vi "JanisDC_3Channel_LKS331_3SRS830.vi"() -> ()   [LabVIEW 2014]
uses:
  <vilib>/Utility/file.llb/Write To Spreadsheet File (DBL).vi
panel:
  out "Probe Temp":dbl format="%.3f"
  out "Cryostat Temp":dbl format="%.3f"
  in  "Tab Control":enum32{"Page 1", "Page 3"}(tab)
  in  "Start T":dbl=130.0
  in  "T Step":dbl=1.0
  in  "End T":dbl
  in  "Mid T":dbl
  in  "T Step 2":dbl=1.0
  in  "Seconds for Stability":dbl=200.0
  in  "SRS830_1\nAddress":i16
  in  "SRS830_2\nAddress":i16
  in  "Save file path":path
  in  "error in (no error)":errorcluster
  out "error out":errorcluster
  in  "Amplitude":dbl=0.75
  in  "Delay Time (s)":dbl=0.4
  in  "Frequency":dbl=0.1
  in  "Offset":dbl=3.0
  in  "Phase":dbl
  in  "Amplifier Offset":dbl=0.1 caption="Frequency"
  in  "Amplifier Gain":dbl=0.1 caption="Frequency"
  in  "LKS331\nAddress":i16
  in  "Setpoint Proximity":dbl=0.01 format="%#.3g"
  in  "Required Stability":dbl=0.002 format="%#.4g"
  in  "SRS830_3\nAddress":i16
  out "XY Graph 3":cluster{dbl, dbl}[](graph) caption="SRS2"
  out "XY Graph 4":cluster{dbl, dbl}[](graph) caption="SRS1"
  out "XY Graph 5":cluster{dbl, dbl}[](graph) caption="LR700"
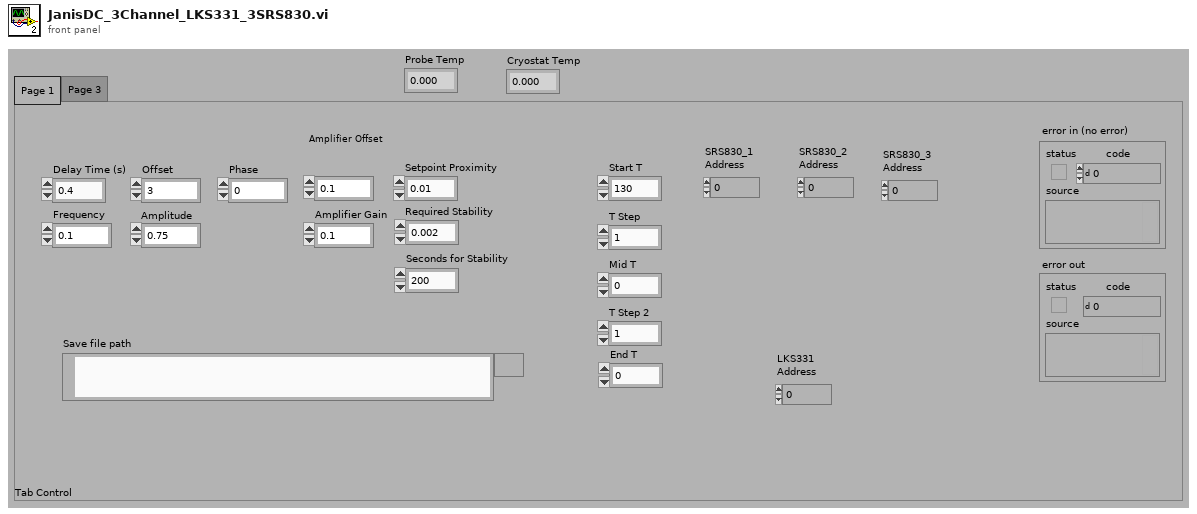
[diagram p1: front panel]
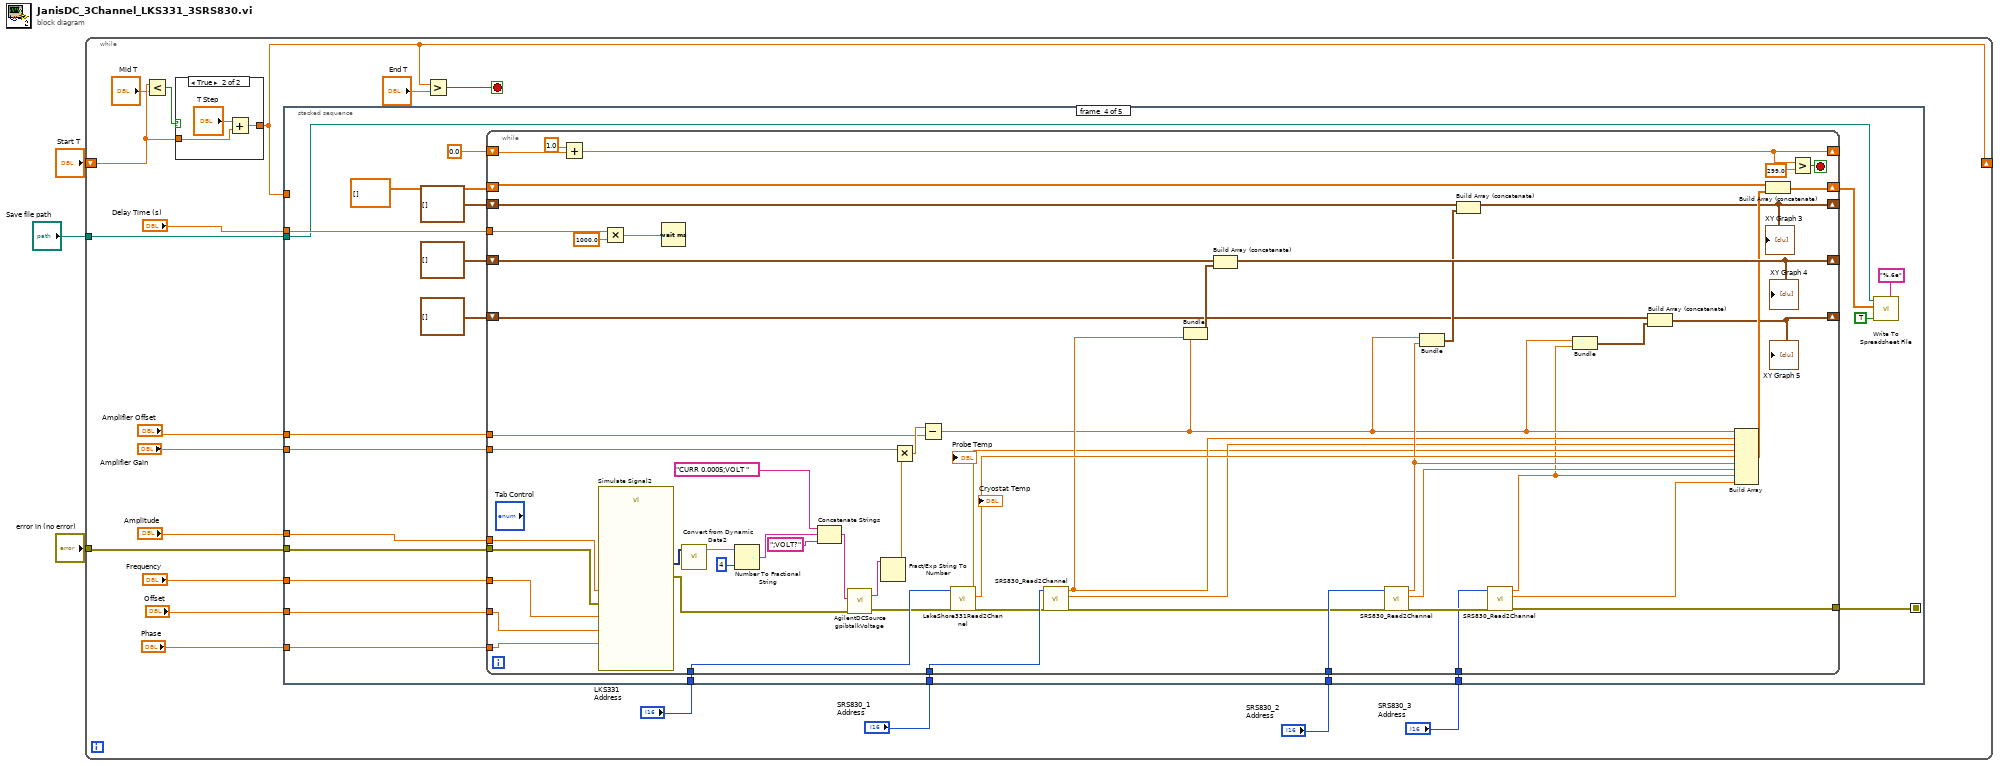
[diagram p0: block diagram]
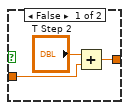
[diagram p2: hidden frame]
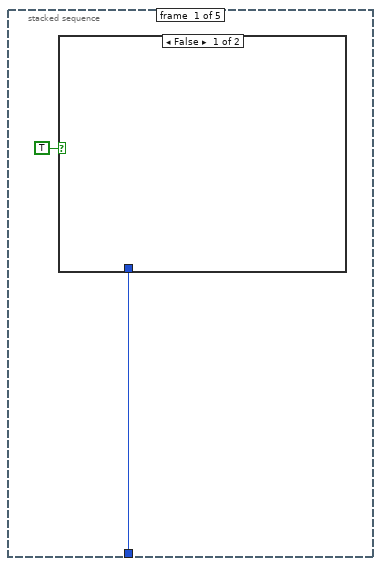
[diagram p3: hidden frame]
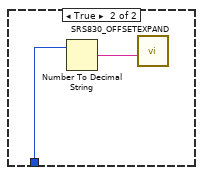
[diagram p4: hidden frame]
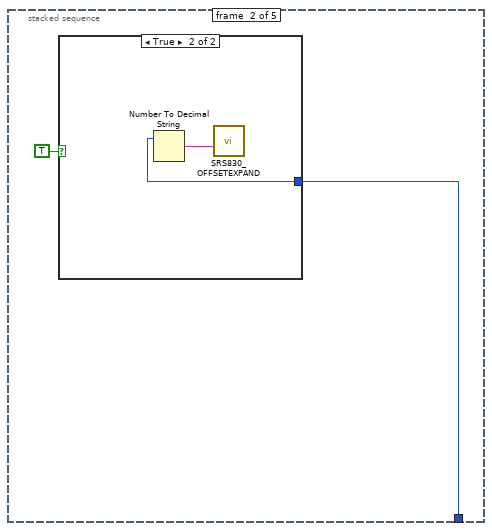
[diagram p5: hidden frame]
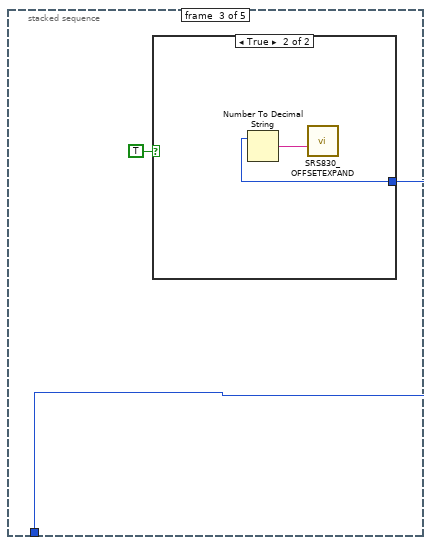
[diagram p7: hidden frame]
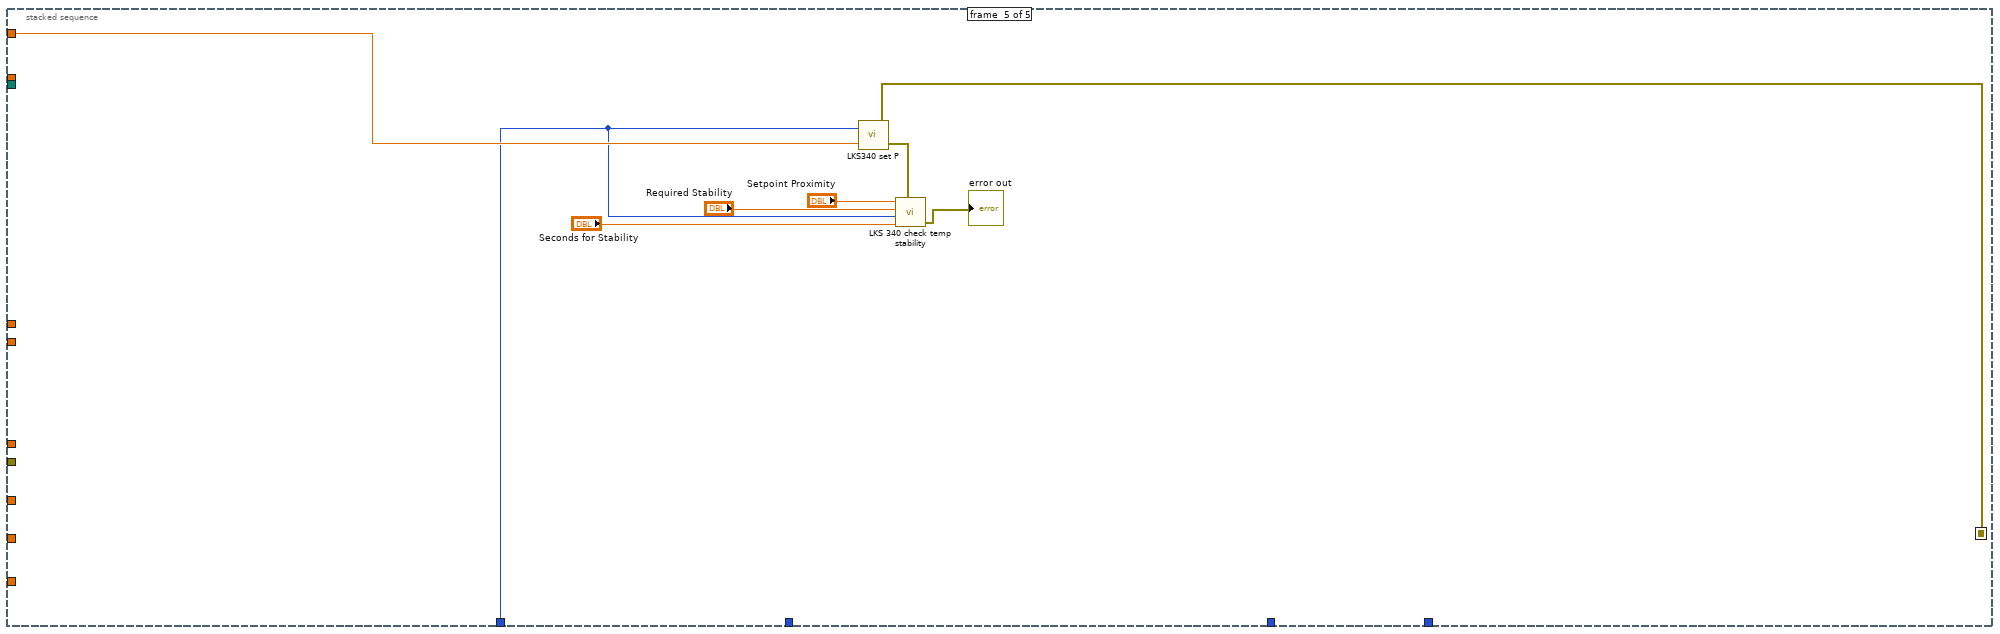
[diagram p9: hidden frame]
diagram:
  n1 = while {
    shift-right: [w17] -> _
    shift-left: "Start T" -> [w20]
    tunnel: "error in (no error)" -> [w16]
    tunnel: "Save file path" -> [w6]
    stop <- w22 stop-if-true
    n2 = Less?(x=w20, y="Mid T") -> (x < y?=w21:bool)
    n3 = case shown="True" w21 {
      tunnel: w20 -> [w24 w27]
      tunnel: [w23 w26] -> w17
      frame False {
        n4 = Add(x="T Step 2", y=w24) -> (x+y=w23:dbl)
      }
      frame True {
        n5 = Add(x="T Step", y=w27) -> (x+y=w26:dbl)
      }
    }
    n6 = stacked-sequence {
      seq-local: [_ _ _ w58 _] -> [_ _ _ _ w119]
      tunnel: w17 -> [_ _ _ _ w126]
      tunnel: w16 -> [_ _ _ w59 _]
      tunnel: "SRS830_1\nAddress" -> [w30 _ _ w56 _]
      tunnel: "SRS830_2\nAddress" -> [_ w34 _ w55 _]
      tunnel: "Amplitude" -> [_ _ _ w54 _]
      tunnel: "Frequency" -> [_ _ _ w53 _]
      tunnel: "Offset" -> [_ _ _ w52 _]
      tunnel: "Phase" -> [_ _ _ w51 _]
      tunnel: "Delay Time (s)" -> [_ _ _ w50 _]
      tunnel: "Amplifier Gain" -> [_ _ _ w49 _]
      tunnel: "Amplifier Offset" -> [_ _ _ w48 _]
      tunnel: w6 -> [_ _ _ w44 _]
      tunnel: "LKS331\nAddress" -> [_ _ _ w43 w120]
      tunnel: "SRS830_3\nAddress" -> [_ _ w37 w41 _]
      frame #0 {
        n7 = case shown="False" TRUE {
          tunnel: w30 -> [_ w31]
          frame False {
          }
          frame True {
            n8 = Number To Decimal String(number=w31) -> (decimal integer string=w32:string)  [unwired: 1 in]
            n9 = call "SRS830_OFFSETEXPAND.vi"("address string"=w32) -> ()  [unwired: 11 in]
          }
        }
      }
      frame #1 {
        n10 = case shown="True" TRUE {
          tunnel: w34 -> [_ w35]
          frame False {
          }
          frame True {
            n11 = Number To Decimal String(number=w35) -> (decimal integer string=w36:string)  [unwired: 1 in]
            n12 = call "SRS830_OFFSETEXPAND.vi"("address string"=w36) -> ()  [unwired: 11 in]
          }
        }
      }
      frame #2 {
        n13 = case shown="True" TRUE {
          tunnel: w37 -> [_ w39]
          frame False {
          }
          frame True {
            n14 = Number To Decimal String(number=w39) -> (decimal integer string=w40:string)  [unwired: 1 in]
            n15 = call "SRS830_OFFSETEXPAND.vi"("address string"=w40) -> ()  [unwired: 11 in]
          }
        }
      }
      frame #3 {
        n16 = while {
          shift-right: [w111] -> _
          shift-left: cluster{dbl, dbl}[] [] -> [w97]
          shift-right: [w109] -> w45
          shift-left: dbl[][] [] -> [w110]
          shift-right: [w105] -> _
          shift-left: 0.0 -> [w108]
          tunnel: w59 -> [w100]
          tunnel: [w66] -> w58
          shift-right: [w85] -> _
          shift-left: cluster{dbl, dbl}[] [] -> [w95]
          tunnel: w56 -> [w82]
          tunnel: w55 -> [w81]
          tunnel: w54 -> [w92]
          tunnel: w53 -> [w91]
          tunnel: w52 -> [w90]
          tunnel: w51 -> [w89]
          tunnel: w50 -> [w88]
          tunnel: w49 -> [w87]
          tunnel: w48 -> [w74]
          tunnel: w43 -> [w84]
          shift-right: [w72] -> _
          shift-left: cluster{dbl, dbl}[] [] -> [w71]
          tunnel: w41 -> [w65]
          stop <- w106 stop-if-true
          n17 = Add(x=1.0, y=w108) -> (x+y=w105:dbl)
          n18 = call "Simulate Signal2"("Offset"=w90, "Frequency"=w91, "Amplitude"=w92, "Phase"=w89, "error in (no error)"=w100) -> ("Triangle"=w118:dynamicdata, "error out"=w99:errorcluster)  [unwired: 9 in]
          n19 = Multiply(x=w88, y=1000.0) -> (x*y=w102:dbl)
          n20 = Wait (ms)(milliseconds to wait=w102) -> ()  [unwired: 1 out]
          n21 = call "Convert from Dynamic Data2"("Dynamic Data Type"=w118) -> ("Scalar"=w117:dbl)  [unwired: 3 in]
          n22 = Number To Fractional String(number=w117, precision (6)=4) -> (F-format string=w116:string)  [unwired: 2 in]
          n23 = Concatenate Strings("CURR 0.0005;VOLT ", w116, ";VOLT?") -> (w112:string)
          n24 = call "AgilentDCSource gpibtalkVoltage.vi"("error in"=w99, "Send"=w112) -> ("error out"=w83:errorcluster, "read"=w93:string)  [unwired: 2 in]
          n25 = Fract/Exp String To Number(string=w93) -> (number=w94:dbl)  [unwired: 3 in, 1 out]
          n26 = Multiply(x=w87, y=w94) -> (x*y=w101:dbl)
          n27 = Subtract(x=w101, y=w74) -> (x-y=w69:dbl)
          n28 = call "LakeShore331Read2Channel.vi"("error in (no error)"=w83, "LKS331\nGPIB Address"=w84) -> ("error out"=w80:errorcluster, "TempCryostat"=w78:dbl, "TempProbe"=w68:dbl)  [unwired: 7 in]
          "Cryostat Temp" <- w78
          "Probe Temp" <- w68
          n29 = call "SRS830_Read2Channel.vi"("error in (no error)"=w80, "Lock in\nGPIB Address"=w82) -> ("error out"=w79:errorcluster, "Ch_OUTP3"=w73:dbl, "Ch_OUTR1"=w75:dbl)  [unwired: 7 in]
          n30 = Bundle(w69, "Ch_OUTR1"=w75) -> (w96:cluster{dbl, "Ch_OUTR1":dbl})  [unwired: 1 in]
          n31 = Build Array (concatenate)(w97, w96) -> (w111:cluster{dbl, "Ch_OUTR1":dbl}[])
          "XY Graph 4" <- w111
          n32 = call "SRS830_Read2Channel.vi"("error in (no error)"=w79, "Lock in\nGPIB Address"=w81) -> ("error out"=w67:errorcluster, "Ch_OUTP3"=w76:dbl, "Ch_OUTR1"=w77:dbl)  [unwired: 7 in]
          n33 = Bundle(w69, "Ch_OUTR1"=w77) -> (w98:cluster{dbl, "Ch_OUTR1":dbl})  [unwired: 1 in]
          n34 = Build Array (concatenate)(w95, w98) -> (w85:cluster{dbl, "Ch_OUTR1":dbl}[])
          "XY Graph 3" <- w85
          n35 = call "SRS830_Read2Channel.vi"("error in (no error)"=w67, "Lock in\nGPIB Address"=w65) -> ("error out"=w66:errorcluster, "Ch_OUTP3"=w64:dbl, "Ch_OUTR1"=w63:dbl)  [unwired: 7 in]
          n36 = Bundle(w69, "Ch_OUTR1"=w63) -> (w70:cluster{dbl, "Ch_OUTR1":dbl})  [unwired: 1 in]
          n37 = Build Array (concatenate)(w71, w70) -> (w72:cluster{dbl, "Ch_OUTR1":dbl}[])
          "XY Graph 5" <- w72
          n38 = Build Array(w69, w75, w73, w68, w78, w77, w76, w63, w64) -> (w86:dbl[])
          n39 = Build Array (concatenate)(w110, w86) -> (w109:dbl[][])
          n40 = Greater?(x=w105, y=299.0) -> (0:w106:bool)
        }
        n41 = call-poly <vilib>:"Write To Spreadsheet File.vi"("format (%.3f)"="%.6e", "append to file? (new file:F)"=TRUE, "2D data"=w45, "file path (dialog if empty)"=w44) -> ()  [unwired: 4 in, 1 out]
      }
      frame #4 {
        n42 = call "LKS340 set P.vi"("error in"=w119, "Set point"=w126, "GPIB Adress"=w120) -> ("error out"=w124:errorcluster)
        n43 = call "LKS 340 check temp stability.vi"("Set point proximity"="Setpoint Proximity", "Stability"="Required Stability", "GPIB Address"=w120, "seconds to wait"="Seconds for Stability", "error in"=w124) -> ("error out"=→"error out":errorcluster)  [unwired: 2 in]
      }
    }
    n44 = Greater?(x=w17, y="End T") -> (0:w22:bool)
  }
